vi "domeADB_getSample_status.vi"(8 "error in (no error)":errorcluster, 11 "status_Ctl":T1={"position_error"=0.0, "position_actual"=0.0, "position_cmd"=0.0, "drive_torque_actual[5]"=[0.0, 0.0, 0.0, 0.0, 0.0], "drive_torque_error[5]"=[0.0, 0.0, 0.0, 0.0, 0.0], "drive_torque_cmd[5]"=[0.0, 0.0, 0.0, 0.0, 0.0], "drive_current_actual[5]"=[0.0, 0.0, 0.0, 0.0, 0.0], "drive_temp_actual[5]"=[0.0, 0.0, 0.0, 0.0, 0.0], "encoder_head_raw[5]"=[0.0, 0.0, 0.0, 0.0, 0.0], "encoder_head_calibrated[5]"=[0.0, 0.0, 0.0, 0.0, 0.0], "resolver_raw[5]"=[0.0, 0.0, 0.0, 0.0, 0.0], "resolver_calibrated[5]"=[0.0, 0.0, 0.0, 0.0, 0.0]}) -> (0 "error out":errorcluster, 2 "function return":i32, 3 "status_Ctl out":T1)   [LabVIEW 2016, in "SALLV_domeADB.lvlib"]
doc: "int domeADB_shm_getSample_statusLV(domeADB_statusLV *status_Ctl );"
uses:
  SALLV_domeADB.lvlib
  DataTypes/status.ctl
  SALLV_domeADB.so
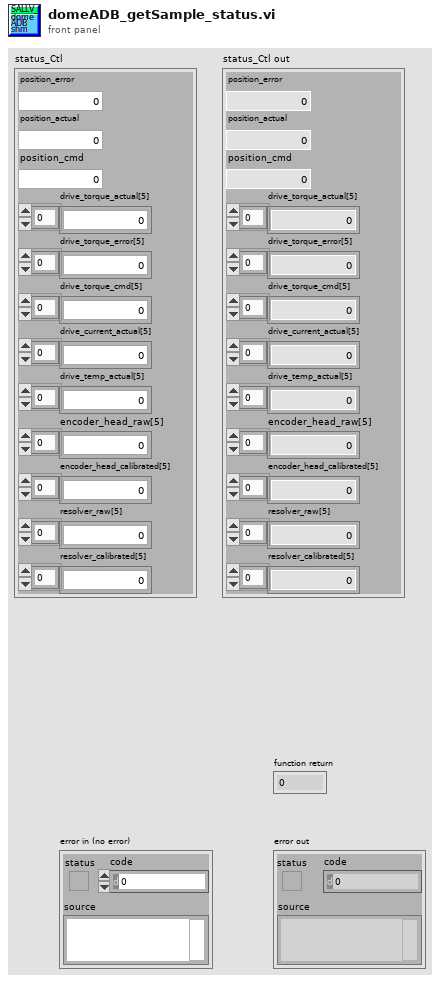
[diagram p1: front panel]
types:
  T1 = typedef "SALLV_domeADB.lvlib/status.ctl" = cluster{"position_error":sgl, "position_actual":sgl, "position_cmd":sgl, "drive_torque_actual[5]":sgl[], "drive_torque_error[5]":sgl[], "drive_torque_cmd[5]":sgl[], "drive_current_actual[5]":sgl[], "drive_temp_actual[5]":sgl[], "encoder_head_raw[5]":sgl[], "encoder_head_calibrated[5]":sgl[], "resolver_raw[5]":sgl[], "resolver_calibrated[5]":sgl[]}
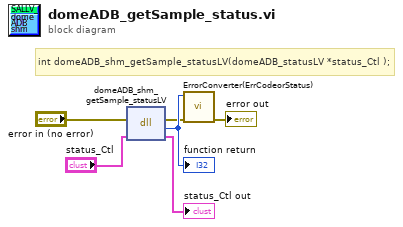
[diagram p0: block diagram]
diagram:
  # "int domeADB_shm_getSample_statusLV(domeADB_statusLV *status_Ctl );"
  n1 = dll-call lib="home/andres/Desktop/SALLV_domeADB/SALLV_domeADB.*" fn="domeADB_shm_getSample_statusLV"(error in="error in (no error)", "status_Ctl"="status_Ctl") -> (error out=w2:errorcluster, w6:i32, "status_Ctl"=→"status_Ctl out":T1)  [unwired: 2 in, 1 out]
  "function return" <- w6
  n2 = call "ErrorConverter(ErrCodeorStatus).vi"("error in (no error)"=w2, "error code"=w6) -> ("error out"=→"error out":errorcluster)  [unwired: 9 in]
